vi "Agilent ENA Series Thru Response Calibration.vi"() -> ()   [LabVIEW 2020]
doc: "Performs thru calibration between two ports. The default configuration is S12 calibration."
uses:
  <instrlib>/Agilent ENA Series/Agilent ENA Series.lvlib
panel:
  in  "Port 2 - stimulus (2)":i32=2
  in  "Port 1 - response (1)":i32=1
  in  "VISA resource name":refnum<visa-resource-name>
  # "(c) 2005-2021 National Instruments.  ALL RIGHTS RESERVED."
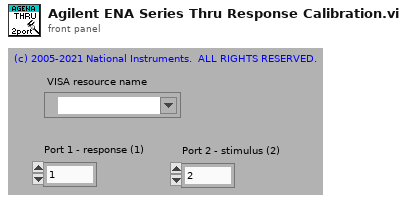
[diagram p1: front panel]
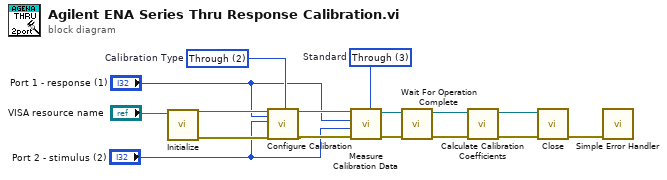
[diagram p0: block diagram]
diagram:
  w3 = u16 2 items=["Open", "Short", "Through", "1-port", "Full 2-port", "Full 3-port", "Full 4-port", "Enhanced Response", "Gain Phase Open", "Gain Phase Short", "Gain Phase Through", "Gain Phase 1 port "]  # Calibration Type
  w14 = u16 3 items=["Open", "Short", "Load", "Through", "Isolation", "Gain Phase Open", "Gain Phase Short", "Gain Phase Load", "Gain Phase Through", "Gain Phase Isolation"]  # Standard
  n1 = call <instrlib>:"Initialize.vi"("VISA resource name"="VISA resource name") -> ("error out"=w13:errorcluster, "VISA resource name out"=w11:refnum<visa-resource-name>)  [unwired: 9 in]
  n2 = call <instrlib>:"Configure Calibration.vi"("VISA resource name"=w11, "Port 1 (1)"="Port 1 - response (1)", "Port 2 (1)"="Port 2 - stimulus (2)", "error in (no error)"=w13, "Calibration Type (6: Full 4-port)"=w3) -> ("VISA resource name out"=w10:refnum<visa-resource-name>, "error out"=w12:errorcluster)  [unwired: 13 in]
  n3 = call <instrlib>:"Measure Calibration Data.vi"("Standard (0: Open)"=w14, "error in (no error)"=w12, "Port 2 - stimulus (2)"="Port 2 - stimulus (2)", "Port 1 - response (1)"="Port 1 - response (1)", "VISA resource name"=w10) -> ("error out"=w9:errorcluster, "VISA resource name out"=w8:refnum<visa-resource-name>)  [unwired: 5 in]
  n4 = call <instrlib>:"Wait For Operation Complete.vi"("error in (no error)"=w9, "VISA resource name"=w8) -> ("error out"=w7:errorcluster, "VISA resource name out"=w5:refnum<visa-resource-name>)  [unwired: 8 in]
  n5 = call <instrlib>:"Calculate Calibration Coefficients.vi"("error in (no error)"=w7, "VISA resource name"=w5) -> ("error out"=w6:errorcluster, "VISA resource name out"=w4:refnum<visa-resource-name>)  [unwired: 8 in]
  n6 = call <instrlib>:"Close.vi"("error in (no error)"=w6, "VISA resource name"=w4) -> ("error out"=w15:errorcluster)  [unwired: 9 in]
  n7 = call <vilib>:"Simple Error Handler.vi"("error in (no error)"=w15) -> ()  [unwired: 4 in, 5 out]
